vi "Write Context.vi"(8 "error in (no error)":errorcluster, 10 "Context":refnum<vi>, 11 "PLC_Module in":refnum<class "PLC_Module.lvclass">) -> (0 "error out":errorcluster, 3 "PLC_Module out":refnum<class "PLC_Module.lvclass">)   [LabVIEW 2025, in "PLC_Module.lvlib" / "PLC_Module.lvclass"]
uses:
  PLC_Module.lvclass
  PLC_Module.lvclass/PLC_Module.ctl
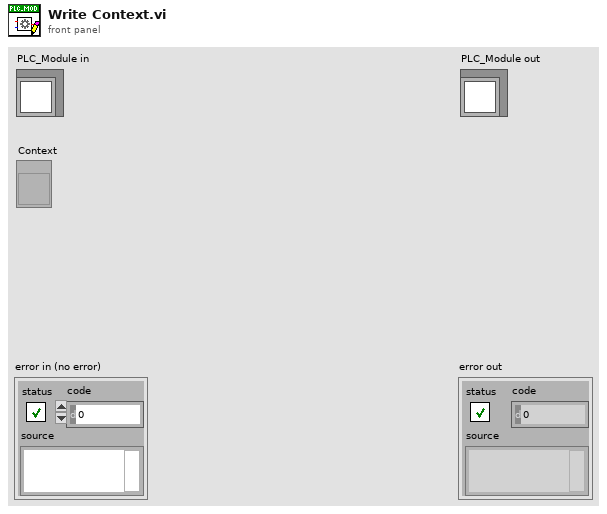
[diagram p1: front panel]
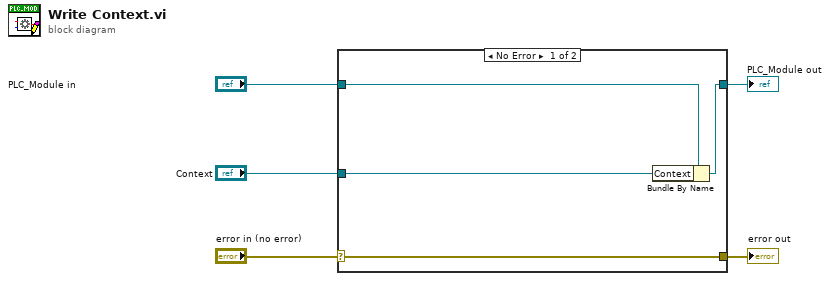
[diagram p0: block diagram]
diagram:
  n1 = case shown="No Error" "error in (no error)" {
    selector: "error in (no error)" -> [w9 w10]
    tunnel: [w9 w10] -> w4
    tunnel: [w7 w11] -> w2
    tunnel: "PLC_Module in" -> [w8 w11]
    tunnel: "Context" -> [w6 _]
    frame No Error {
      n2 = Bundle By Name(cluster=w8, "Context"=w6) -> (w7:refnum<class "PLC_Module.lvclass">)
    }
    frame Error {
    }
  }
  "error out" <- w4
  "PLC_Module out" <- w2
